vi "X10468 SLM Make Tophat.vi"(0 "R Array":dbl[][](array[numeric]), 11 "Normalized Radius":dbl) -> (8 "Tophat Holo":dbl[][](array[numeric]))   [LabVIEW 2018]
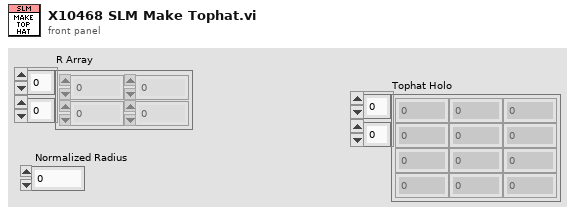
[diagram p1: front panel]
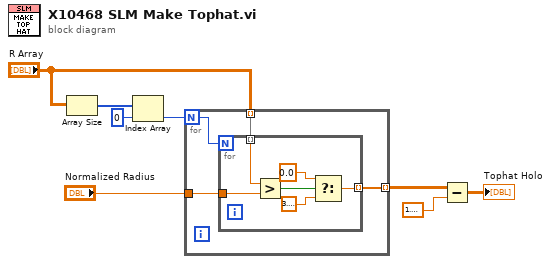
[diagram p0: block diagram]
diagram:
  n1 = Array Size(array="R Array") -> (size(s)=w8:i32[])
  n2 = Index Array(array=w8, index=0) -> (element=w6:i32)
  n3 = for {
    N: w6 -> [w12]
    tunnel: "Normalized Radius" -> [w11]
    tunnel: [w10] -> w3 mode=indexing
    tunnel: "R Array" -> [w9] mode=indexing
    n4 = for {
      N: w12 -> [_]
      tunnel: w11 -> [w18]
      tunnel: [w14] -> w10 mode=indexing
      tunnel: w9 -> [w13] mode=indexing
      n5 = Greater?(x=w13, y=w18) -> (0:w17:bool)
      n6 = Select(t=0.0, s=w17, f=3.141592653589793) -> (s? t:f=w14:dbl)
    }
  }
  n7 = Subtract(x=w3, y=1.5707963267948966) -> (x-y=→"Tophat Holo":dbl[][])
